vi "Change Default Value.vi"(8 "Error In":errorcluster, 9 "New Default Values":dbl[](array[numeric]), 10 "Channels":string[](array[string]), 11 "System Definition Path":path=path "C:/Users/Public/Documents/National Instruments/NI VeriStand 2013/Projects/Untitled 3/Untitled 3.nivssdf") -> (0 "error out":errorcluster)   [LabVIEW 2012]
uses:
  NationalInstruments.VeriStand.SystemDefinitionAPI
  NationalInstruments.VeriStand.SystemStorage
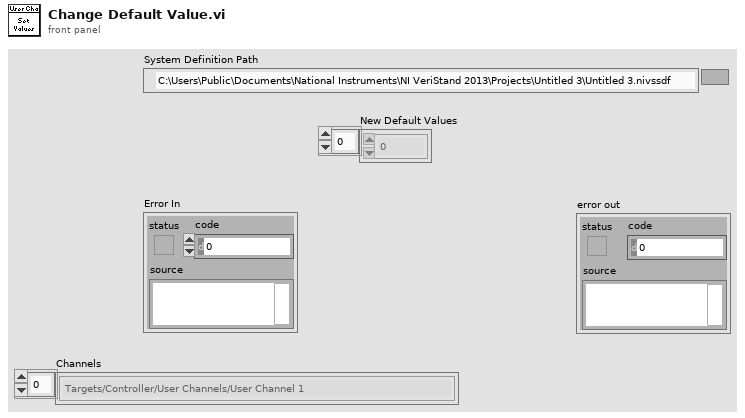
[diagram p1: front panel]
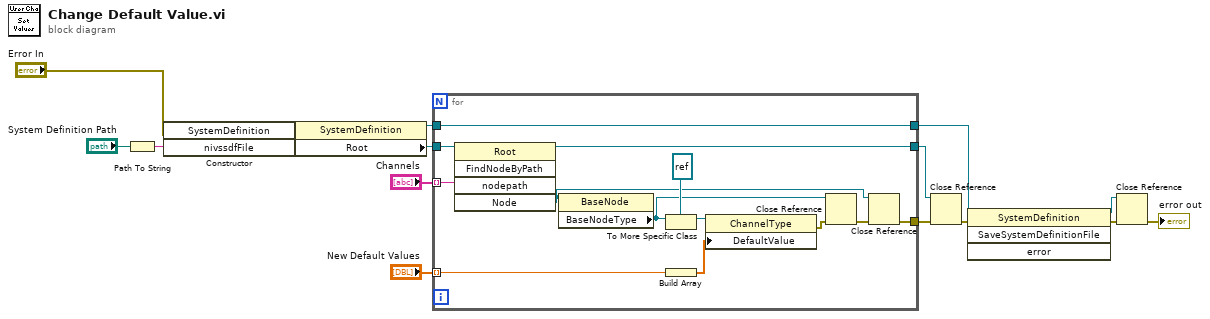
[diagram p0: block diagram]
diagram:
  n1 = Path To String(path="System Definition Path") -> (string=w16:string)
  n2 = constructor class="SystemDefinition"(error in="Error In", "nivssdfFile"=w16) -> (reference out=w10:refnum<k24>, error out=w12:errorcluster)  [unwired: 2 in, 2 out]
  n3 = property class="SystemDefinition"(reference=w10, error in=w12) -> (reference out=w9:refnum<k24>, "Root"=w11:refnum<k24>)  [unwired: 1 out]
  n4 = for {
    tunnel: w11 -> [w29]
    tunnel: "New Default Values" -> [w25] mode=indexing
    tunnel: w9 -> [w17]
    tunnel: "Channels" -> [w28] mode=indexing
    tunnel: [w18] -> w4
    tunnel: [w19] -> w3
    tunnel: [w17] -> w2
    n5 = invoke class="Root" method="FindNodeByPath"(reference=w29, "nodepath"=w28) -> (reference out=w19:refnum<k24>, "Node"=w20:refnum<k24>)  [unwired: 3 in, 3 out]
    n6 = property class="BaseNode"(reference=w20) -> ("BaseNodeType"=w22:refnum<k24>)  [unwired: 1 in, 2 out]
    n7 = To More Specific Class(target class=refnum<k24> refnum ("reference out"), reference=w22) -> (specific class reference=w27:refnum<k24>)  [unwired: 1 in, 1 out]
    n8 = Build Array(w25) -> (w24:dbl[])
    n9 = property class="ChannelType"(reference=w27, "DefaultValue"=w24) -> (error out=w23:errorcluster)  [unwired: 1 in, 1 out]
    n10 = Close Reference(reference=w22, error in (no error)=w23) -> (error out=w21:errorcluster)
    n11 = Close Reference(reference=w20, error in (no error)=w21) -> (error out=w18:errorcluster)
  }
  n12 = Close Reference(reference=w3, error in (no error)=w4) -> (error out=w5:errorcluster)
  n13 = invoke class="SystemDefinition" method="SaveSystemDefinitionFile"(reference=w2, error in=w5) -> (reference out=w8:refnum<k24>, error out=w7:errorcluster)  [unwired: 2 in, 2 out]
  n14 = Close Reference(reference=w8, error in (no error)=w7) -> (error out=→"error out":errorcluster)
